vi "VM_ProjetoV5.3.vi"() -> ()   [LabVIEW 2016, in "Projeto_Modbus_Finalizado.lvlib"]
uses:
  Projeto_Modbus_Finalizado.lvlib
  <vilib>/userdefined/High Color/IMAQdx.ctl
  <vilib>/Analysis/baseanly.llb/Mean (DBL).vi
  <vilib>/lvdsc/process/Deploy Library.vi
  <vilib>/Utility/file.llb/Read Delimited Spreadsheet (DBL).vi
  <vilib>/Utility/file.llb/Write Delimited Spreadsheet (DBL).vi
  <vilib>/lvdsc/process/Undeploy Library.vi
  <vilib>/vision/driver/NI_Vision_Acquisition_Software.lvlib
  <resource>/objmgr/imaqdx.rc
  <vilib>/Analysis/NI_AALBase.lvlib
  <vilib>/lvdsc/NI_DSC.lvlib
panel:
  in  "Reset Game":bool
  in  "Reset Count":bool
  out "GameOver":bool
  out "y place":dbl
  out "x place":dbl
  out "pick angle":dbl
  out "place angle":dbl
  out "y pick":dbl
  out "x pick":dbl
  in  "Calibração\nRobô":path=path "C:/Users/rodrigorg1/Desktop/Projeto/calibracaoRobo.csv"
  in  "Calibração\nMesa":path=path "C:/Users/rodrigorg1/Desktop/Projeto/calibracaoMesa.csv"
  out "Error Out":errorcluster
  in  "Cut Limit":dbl=65.0 format="%#_13g"
  in  "Confirma":bool
  out "Status":string
  out "Câmera Robo":T1(plugin-control)
  out "Câmera Mesa":T1(plugin-control)
  in  "Começa jogada":bool
  in  "stop":bool
  in  "Source Câmera Robo":T2="S1156978"
  in  "Source Câmera Mesa":T2="cam0"
  out "Dobrao":bool
  out "Passa Vez":bool
  # "x 91\ny 176"
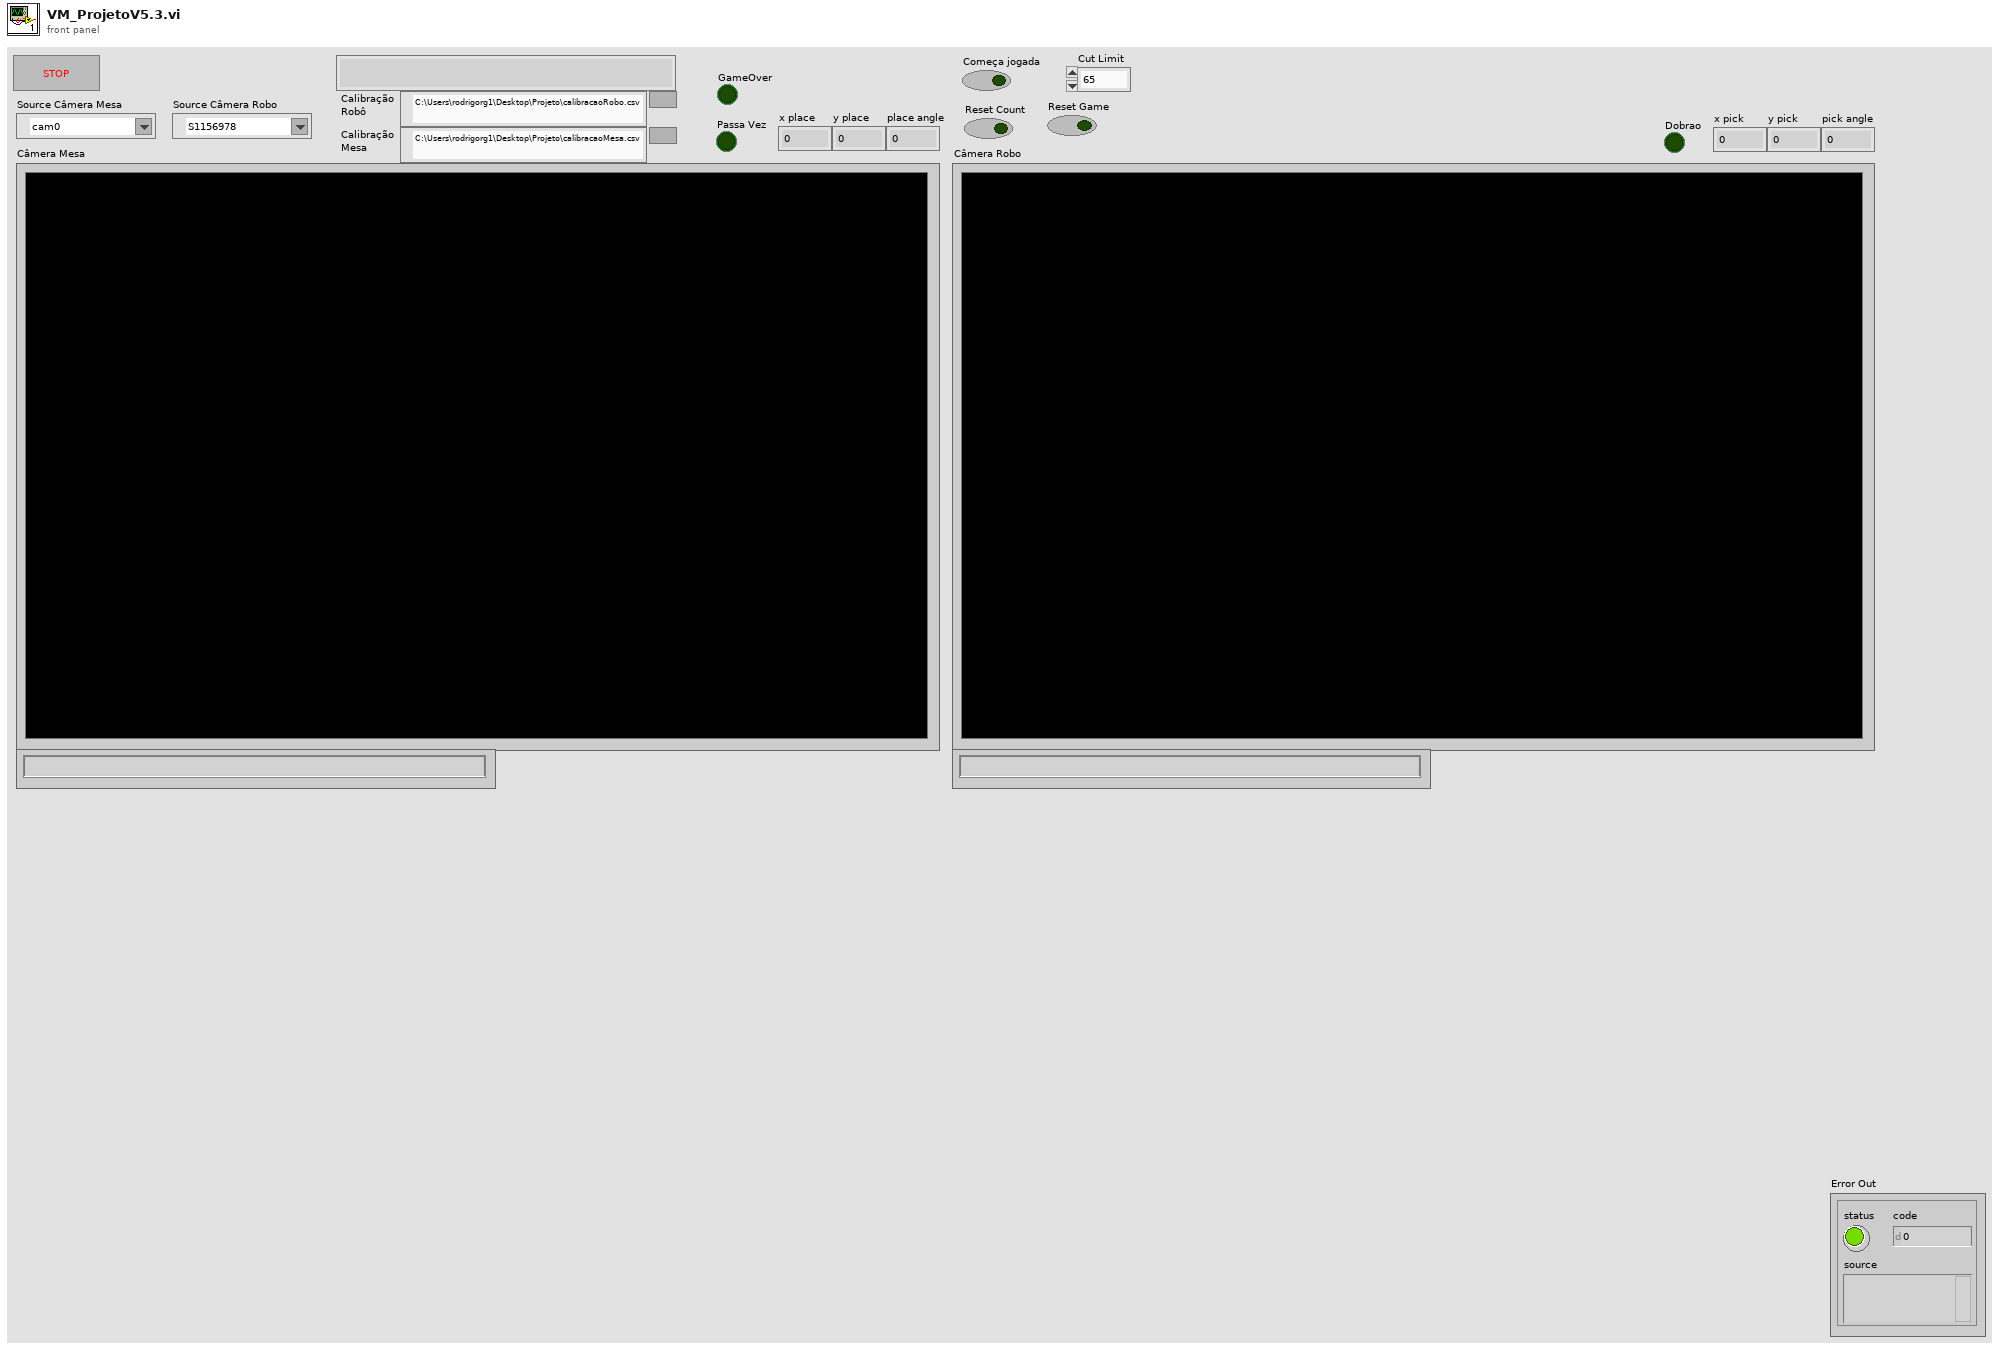
[diagram p1: front panel]
types:
  T1 = typedef "IMAQ Image.ctl" = refnum<image>
  T2 = typedef "IMAQdx.ctl" = refnum<k21>
  T3 = typedef "IMAQ Rectangle" = cluster{"Left":i32, "Top":i32, "Right":i32, "Bottom":i32, "Rotation":dbl}
  T4 = typedef "ROI Descriptor" = cluster{"Global Rectangle":i32[], "Contours":cluster{"ID":enum32{"External", "Internal"}, "Type":u32, "Coordinates":i32[]}[]}
  T5 = cluster{"Position":cluster{"x":sgl, "y":sgl}, "Angle":sgl, "Scale":sgl, "Score":sgl, "Bounding Box":cluster{"x":sgl, "y":sgl}[]}[]
  T6 = cluster{"Centro Peça":dbl[], "Centros Númeors":dbl[][], "Números":u8[], "ROI Números":T4[]}[]
  T7 = cluster{"Centro Peça":dbl[], "Centros Númeors":dbl[][], "Números":u8[], "ROI Números":T4[]}
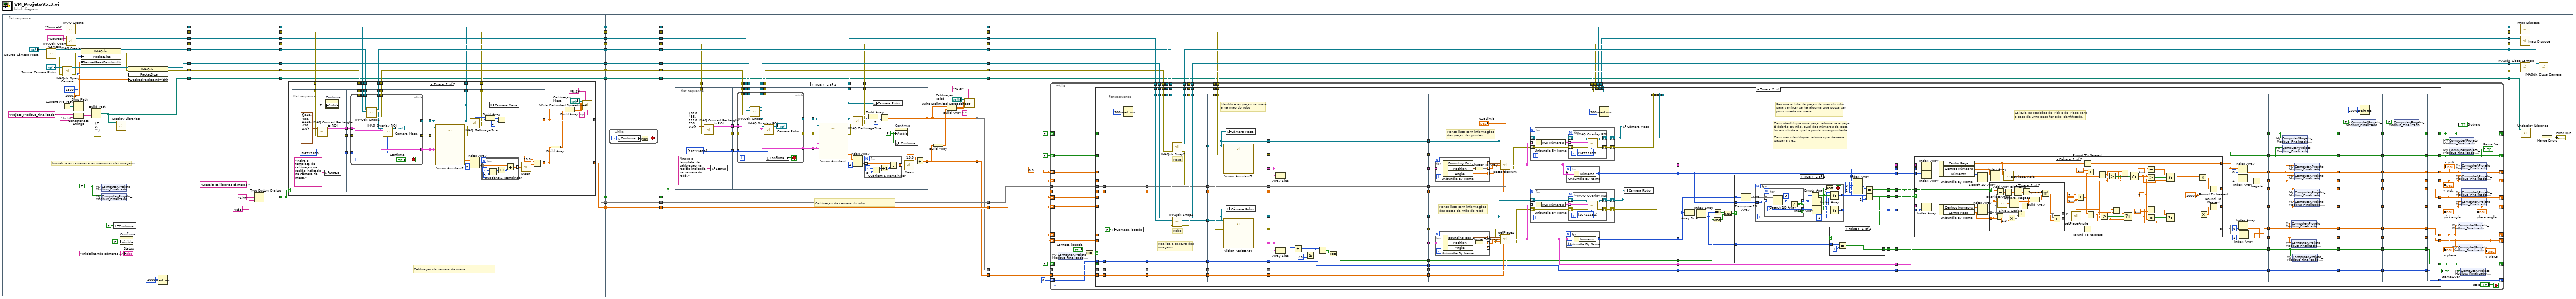
[diagram p0: block diagram]
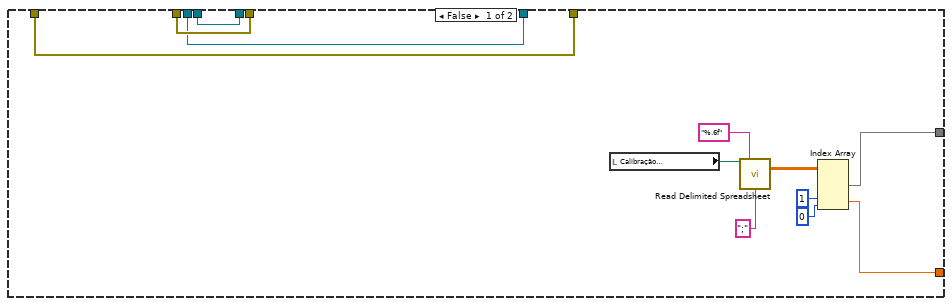
[diagram p2: hidden frame]
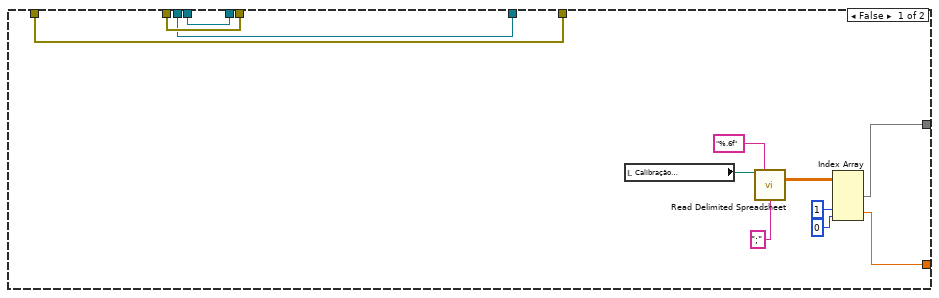
[diagram p3: hidden frame]
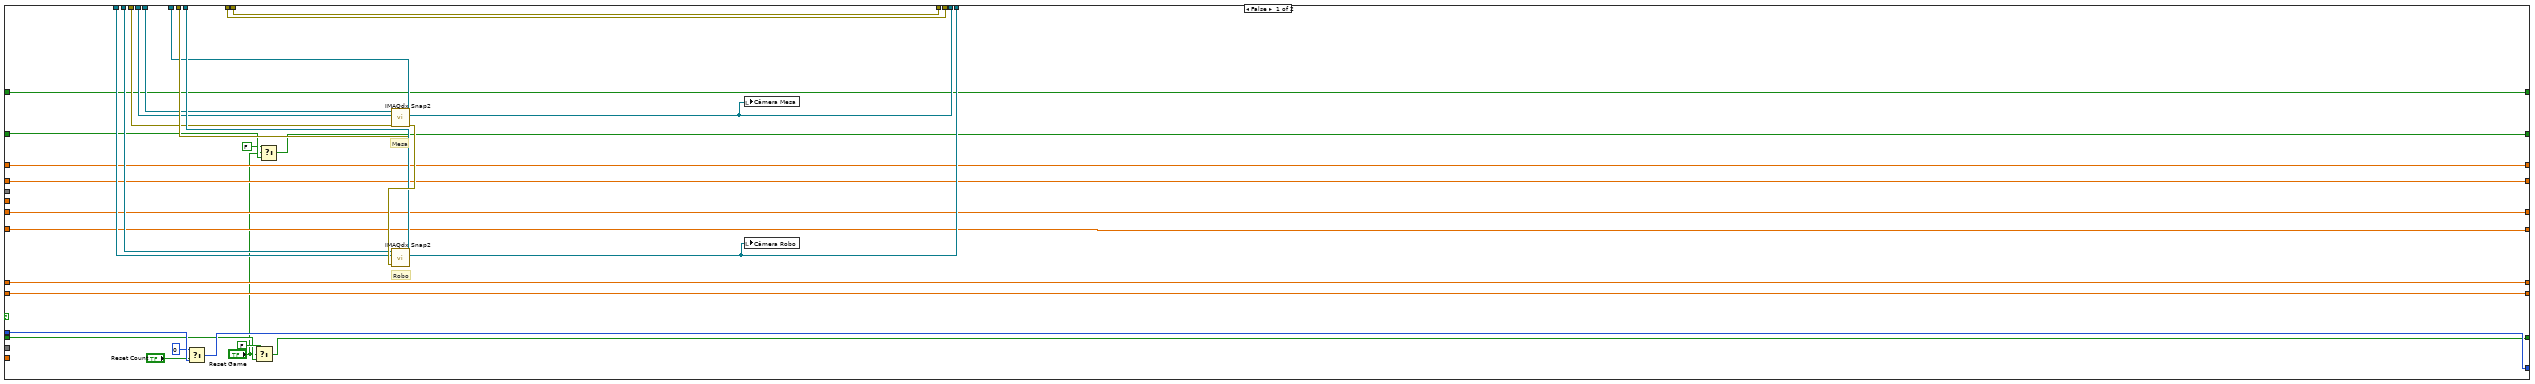
[diagram p4: hidden frame]
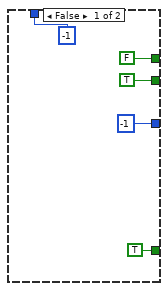
[diagram p5: hidden frame]
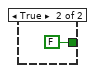
[diagram p6: hidden frame]
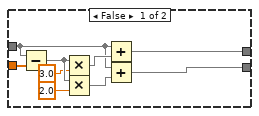
[diagram p7: hidden frame]
diagram:
  n1 = flat-sequence {
    tunnel: [w85] -> w17
    tunnel: [w84] -> w15
    tunnel: [w79] -> w13
    tunnel: [w83] -> w11
    tunnel: [w82] -> w9
    tunnel: [w78] -> w7
    tunnel: [w69] -> w5
    tunnel: [w61] -> w3
    tunnel: w17 -> [w101]
    tunnel: [w101] -> w16
    tunnel: w15 -> [w100]
    tunnel: [w100] -> w14
    tunnel: w13 -> [w99]
    tunnel: [w99] -> w12
    tunnel: w11 -> [w98]
    tunnel: [w98] -> w10
    tunnel: w9 -> [w97]
    tunnel: [w97] -> w8
    tunnel: w7 -> [w96]
    tunnel: [w96] -> w6
    tunnel: w5 -> [w95]
    tunnel: [w95] -> w4
    tunnel: w3 -> [w94]
    tunnel: [w94] -> w2
    tunnel: [w90] -> w1
    tunnel: w16 -> [w115]
    tunnel: w14 -> [w116]
    tunnel: w12 -> [w105]
    tunnel: w10 -> [w114]
    tunnel: w8 -> [w113]
    tunnel: w6 -> [w104]
    tunnel: [w109] -> w41
    tunnel: [w108] -> w39
    tunnel: [w114] -> w37
    tunnel: [w113] -> w35
    tunnel: [w112] -> w33
    tunnel: [w111] -> w31
    tunnel: w4 -> [w111]
    tunnel: [w110] -> w29
    tunnel: [w107] -> w27
    tunnel: [w106] -> w25
    tunnel: [w103] -> w20
    tunnel: w2 -> [w103]
    tunnel: [w102] -> w19
    tunnel: w1 -> [w102]
    tunnel: w41 -> [w213]
    tunnel: [w213] -> w40
    tunnel: w39 -> [w212]
    tunnel: [w212] -> w38
    tunnel: w37 -> [w211]
    tunnel: [w211] -> w36
    tunnel: w35 -> [w210]
    tunnel: [w210] -> w34
    tunnel: w33 -> [w209]
    tunnel: [w209] -> w32
    tunnel: w31 -> [w208]
    tunnel: [w208] -> w30
    tunnel: w29 -> [w207]
    tunnel: [w207] -> w28
    tunnel: w27 -> [w206]
    tunnel: [w206] -> w26
    tunnel: w25 -> [w205]
    tunnel: [w205] -> w24
    tunnel: [w204] -> w21
    tunnel: w20 -> [w204]
    tunnel: w19 -> [w203]
    tunnel: [w203] -> w18
    tunnel: w40 -> [w232]
    tunnel: [w232] -> w52
    tunnel: w38 -> [w231]
    tunnel: [w231] -> w51
    tunnel: w36 -> [w223]
    tunnel: [w222] -> w50
    tunnel: w34 -> [w221]
    tunnel: [w220] -> w49
    tunnel: w32 -> [w230]
    tunnel: [w230] -> w48
    tunnel: w30 -> [w225]
    tunnel: [w224] -> w47
    tunnel: w28 -> [w227]
    tunnel: [w226] -> w46
    tunnel: w26 -> [w229]
    tunnel: [w229] -> w45
    tunnel: w24 -> [w228]
    tunnel: [w228] -> w44
    tunnel: [w219] -> w43
    tunnel: [w218] -> w42
    tunnel: [w217] -> w22
    tunnel: w21 -> [w217]
    tunnel: w18 -> [w216]
    tunnel: [w339] -> w59
    tunnel: [w342] -> w58
    tunnel: [w336] -> w57
    tunnel: [w341] -> w56
    tunnel: [w340] -> w55
    tunnel: [w338] -> w54
    tunnel: [w337] -> w53
    tunnel: w52 -> [w335]
    tunnel: w51 -> [w334]
    tunnel: w50 -> [w333]
    tunnel: w49 -> [w332]
    tunnel: w48 -> [w331]
    tunnel: w47 -> [w330]
    tunnel: w46 -> [w329]
    tunnel: w45 -> [w327]
    tunnel: w44 -> [w328]
    tunnel: w43 -> [w325]
    tunnel: w42 -> [w326]
    tunnel: [w324] -> w23
    tunnel: w22 -> [w324]
    tunnel: w59 -> [w839]
    tunnel: w58 -> [w837]
    tunnel: w57 -> [w841]
    tunnel: w56 -> [w844]
    tunnel: w55 -> [w843]
    tunnel: w54 -> [w840]
    tunnel: w53 -> [w842]
    tunnel: w23 -> [w834]
    frame #0 {
      w60 = FALSE ("000021")
      w73 = 1000.0 ("DesiredPeakBandwidth")
      w74 = u32 1500 ("PacketSize")
      # "Inicializa as câmeras e as memórias das imagens"
      n2 = call <vilib>:"IMAQdx Open Camera.vi"("Session In"="Source Câmera Mesa") -> ("error out"=w77:errorcluster, "Session Out"=w80:T2)  [unwired: 9 in]
      n3 = Current VI's Path() -> (path=w62:path)
      n4 = call <vilib>:"IMAQdx Open Camera.vi"("error in"=w77, "Session In"="Source Câmera Robo") -> ("error out"=w76:errorcluster, "Session Out"=w81:T2)  [unwired: 8 in]
      n5 = call "IMAQ Create"("Image Name"="SourceM") -> ("New Image"=w85:T1, "error out"=w84:errorcluster)  [unwired: 4 in]
      n6 = call "IMAQ Create"("Image Name"="SourceR") -> ("New Image"=w83:T1, "error out"=w82:errorcluster)  [unwired: 4 in]
      n7 = Strip Path(path=w62) -> (stripped path=w63:path)  [unwired: 1 out]
      n8 = Concatenate Strings("Projeto_Modbus_Finalizado" ("library path"), ".lvlib" ("string")) -> (w66:string)
      n9 = property class="IMAQdx"(reference=w80, error in=w76, "PacketSize"=w74, "DesiredPeakBandwidth"=w73) -> (reference out=w79:T2, error out=w75:errorcluster)
      n10 = Build Path(base path=w63, name or relative path=w66) -> (appended path=w61:path)
      n11 = shared-variable "My Computer\\Projeto_Modbus_Finalizado.lvlib\\000021"(w60) -> ()  [unwired: 1 in, 1 out]
      n12 = shared-variable "My Computer\\Projeto_Modbus_Finalizado.lvlib\\000020"(w60) -> ()  [unwired: 1 in, 1 out]
      n13 = local write "Confirma"(FALSE ("Confirma")) -> ()
      n14 = call-poly <vilib>:"Deploy Libraries.vi"("error in (no error)"=errorcluster {"status"=FALSE, "code"=0, "source"=""}, "library path"=w61) -> ()  [unwired: 7 in, 1 out]
      n15 = property on="Confirma" class="Bool (strict)"("Visible"=FALSE) -> ()  [unwired: 2 in, 2 out]
      n16 = property class="IMAQdx"(reference=w81, error in=w75, "PacketSize"=w74, "DesiredPeakBandwidth"=w73) -> (reference out=w69:T2, error out=w78:errorcluster)
      n17 = Wait (ms)(milliseconds to wait=u32 2000) -> ()  [unwired: 1 out]
      "Status" <- "Inicializando câmeras ..." ("Status")
    }
    frame #1 {
      n18 = Two Button Dialog(message="Deseja calibrar as câmeras?", 1:"Não" ("F button name (\"Cancel\")"), 2:"Sim" ("T button name (\"OK\")")) -> (T button?=w90:bool)
    }
    frame #2 {
      # "Calibração da câmera da mesa"
      n19 = case shown="True" w102 {
        tunnel: w116 -> [w125 w143]
        tunnel: w115 -> [w126 w142]
        tunnel: [w127 w141] -> w112
        tunnel: [w128 w140] -> w110
        tunnel: [w126 w139] -> w109
        tunnel: [w125 w138] -> w108
        tunnel: [w118 w133] -> w107
        tunnel: [w117 w134] -> w106
        tunnel: w105 -> [w127 w137]
        tunnel: w104 -> [w128 w136]
        frame False {
          n20 = local read "Calibração\nMesa"() -> (w124:path)
          n21 = call-poly <vilib>:"Read Delimited Spreadsheet.vi"("file path (dialog if empty)"=w124, "format (%.3f)"="%.6f", "delimiter (\\t)"=";" ("delimiter (\\t)")) -> ("all rows"=w121:dbl[][])  [unwired: 7 in, 5 out]
          n22 = Index Array(array=w121, index (row) #2=1, index (col) #2=0) -> (element #1=w117:dbl[], element #2=w118:dbl)  [unwired: 2 in]
        }
        frame True {
          n23 = flat-sequence {
            tunnel: w143 -> [w154]
            tunnel: [w152] -> w149
            tunnel: [w151] -> w148
            tunnel: [u32[] [16711680] ("Colors (Green)")] -> w147
            tunnel: w137 -> [w167]
            tunnel: w136 -> [w166]
            tunnel: w142 -> [w165]
            tunnel: [w164] -> w141
            tunnel: [w163] -> w140
            tunnel: w149 -> [w162]
            tunnel: w148 -> [w161]
            tunnel: [w160] -> w146
            tunnel: [w159] -> w145
            tunnel: [w158] -> w144
            tunnel: w147 -> [w157]
            tunnel: w146 -> [w196]
            tunnel: w145 -> [w195]
            tunnel: [w187] -> w133
            tunnel: w144 -> [w180]
            tunnel: [w180] -> w139
            tunnel: [w182] -> w138
            tunnel: [w181] -> w134
            frame #0 {
              n24 = call "IMAQ Convert Rectangle to ROI"("error in (no error)"=w154, "Rectangle"=T3 {"Left"=818, "Top"=458, "Right"=1118, "Bottom"=758, "Rotation"=0.0}) -> ("error out"=w152:errorcluster, "ROI Descriptor"=w151:T4)  [unwired: 7 in]
              n25 = local write "Status"("Insira o template de calibração na região indicada na câmera da mesa." ("Status")) -> ()
              n26 = property on="Confirma" class="Bool (strict)"("Visible"=TRUE) -> ()  [unwired: 2 in, 2 out]
            }
            frame #1 {
              n27 = while {
                tunnel: w167 -> [w178]
                tunnel: w166 -> [w177]
                tunnel: w165 -> [w176]
                tunnel: [w175] -> w164
                tunnel: [w174] -> w163
                tunnel: w162 -> [w168]
                tunnel: w161 -> [w171]
                tunnel: [w173] -> w160
                tunnel: [w171] -> w159
                tunnel: [w169] -> w158
                tunnel: w157 -> [w170]
                stop <- "Confirma" stop-if-true
                n28 = call <vilib>:"IMAQdx Snap2.vi"("error in"=w177, "Image In"=w176, "Session In"=w178) -> ("error out"=w174:errorcluster, "Image Out"=w169:T1, "Session Out"=w175:T2)  [unwired: 6 in]
                n29 = call "IMAQ Overlay ROI"("Colors (Green)"=w170, "error in (no error)"=w168, "ROI Descriptor"=w171, "Image"=w169) -> ("error out"=w173:errorcluster, "Image Out"=→"Câmera Mesa":T1)  [unwired: 6 in]
              }
            }
            frame #2 {
              n30 = call "Vision Assistant2"("Image In"=w180, "ROI Descriptor (Adv. Straight Edge 1)"=w195, "ROI Descriptor (Copy of Adv. Straight Edge 1)"=w195, "error in"=w196) -> ("Caliper Results (Caliper 2)"=w194:sgl[][], "error out"=w188:errorcluster)  [unwired: 21 in, 1 out]
              n31 = call "IMAQ GetImageSize"("Image"=w180, "error in (no error)"=w188) -> ("Y Resolution"=w186:i32, "X Resolution"=w185:i32, "error out"=w182:errorcluster)  [unwired: 2 in]
              n32 = Index Array(array=w194, index (col)=2 ("disabled index (col)")) -> (element=w192:sgl[])  [unwired: 1 in]
              n33 = for {
                tunnel: w192 -> [w199] mode=indexing
                tunnel: [w197] -> w191 mode=indexing
                i -> [w202]
                n34 = Quotient & Remainder(x=w202, y=5) -> (x-y*floor(x/y)=w200:i32)  [unwired: 1 out]
                n35 = Increment(x=w200) -> (x+1=w198:i32)
                n36 = Divide(x=w199, y=w198) -> (x/y=w197:sgl)
              }
              n37 = Build Array(w185, w186) -> (w184:i32[])
              n38 = local write "Câmera Mesa"(w180) -> ()
              n39 = Divide(x=w184, y=2) -> (x/y=w181:dbl[])
              n40 = call-poly <vilib>:"Mean.vi"("X"=w191) -> ("mean"=w190:dbl)  [unwired: 1 out]
              n41 = Divide(x=10.0, y=w190) -> (x/y=w187:dbl)
            }
          }
          n42 = Build Array(w133) -> (w132:dbl[])
          n43 = Build Array(w134, w132) -> (w131:dbl[][])
          n44 = call-poly <vilib>:"Write Delimited Spreadsheet.vi"("file path (dialog if empty)"="Calibração\nMesa", "format (%.3f)"="%.6f", "2D data"=w131, "delimiter (\\t)"=";" ("delimiter (\\t)")) -> ()  [unwired: 10 in, 2 out]
        }
      }
    }
    frame #3 {
      n45 = while {
        stop <- w215 stop-if-true
        n46 = local read "Confirma"() -> (w214:bool)
        n47 = Not(x=w214) -> (.not. x?=w215:bool)
      }
    }
    frame #4 {
      # "Calibração da câmera do robô"
      n48 = case shown="True" w216 {
        tunnel: w227 -> [w243 w259]
        tunnel: [w243 w258] -> w226
        tunnel: w225 -> [w244 w257]
        tunnel: [w244 w256] -> w224
        tunnel: w223 -> [w242 w255]
        tunnel: [w242 w254] -> w222
        tunnel: w221 -> [w241 w253]
        tunnel: [w241 w252] -> w220
        tunnel: [w233 w246] -> w219
        tunnel: [w234 w245] -> w218
        frame False {
          n49 = local read "Calibração\nRobô"() -> (w235:path)
          n50 = call-poly <vilib>:"Read Delimited Spreadsheet.vi"("file path (dialog if empty)"=w235, "format (%.3f)"="%.6f", "delimiter (\\t)"=";" ("delimiter (\\t)")) -> ("all rows"=w238:dbl[][])  [unwired: 7 in, 5 out]
          n51 = Index Array(array=w238, index (row) #2=1, index (col) #2=0) -> (element #1=w234:dbl[], element #2=w233:dbl)  [unwired: 2 in]
        }
        frame True {
          n52 = flat-sequence {
            tunnel: w253 -> [w270]
            tunnel: [w269] -> w265
            tunnel: [w268] -> w264
            tunnel: [u32[] [16711680] ("Colors (Green)")] -> w263
            tunnel: w257 -> [w282]
            tunnel: w259 -> [w281]
            tunnel: w255 -> [w280]
            tunnel: [w279] -> w256
            tunnel: [w278] -> w258
            tunnel: w265 -> [w277]
            tunnel: w264 -> [w276]
            tunnel: [w275] -> w262
            tunnel: [w274] -> w261
            tunnel: [w273] -> w260
            tunnel: w263 -> [w272]
            tunnel: w262 -> [w312]
            tunnel: w261 -> [w311]
            tunnel: [w303] -> w246
            tunnel: w260 -> [w296]
            tunnel: [w296] -> w254
            tunnel: [w298] -> w252
            tunnel: [w297] -> w245
            frame #0 {
              n53 = call "IMAQ Convert Rectangle to ROI"("error in (no error)"=w270, "Rectangle"=T3 {"Left"=818, "Top"=458, "Right"=1118, "Bottom"=758, "Rotation"=0.0}) -> ("error out"=w269:errorcluster, "ROI Descriptor"=w268:T4)  [unwired: 7 in]
              n54 = local write "Status"("Insira o template de calibração na região indicada na câmera do robô." ("Status")) -> ()
            }
            frame #1 {
              n55 = while {
                tunnel: w282 -> [w294]
                tunnel: w281 -> [w293]
                tunnel: w280 -> [w292]
                tunnel: [w291] -> w279
                tunnel: [w290] -> w278
                tunnel: w277 -> [w289]
                tunnel: w276 -> [w287]
                tunnel: [w288] -> w275
                tunnel: [w287] -> w274
                tunnel: [w286] -> w273
                tunnel: w272 -> [w285]
                stop <- w283 stop-if-true
                n56 = call <vilib>:"IMAQdx Snap2.vi"("error in"=w293, "Image In"=w292, "Session In"=w294) -> ("error out"=w290:errorcluster, "Image Out"=w286:T1, "Session Out"=w291:T2)  [unwired: 6 in]
                n57 = call "IMAQ Overlay ROI"("Colors (Green)"=w285, "error in (no error)"=w289, "ROI Descriptor"=w287, "Image"=w286) -> ("error out"=w288:errorcluster, "Image Out"=→"Câmera Robo":T1)  [unwired: 6 in]
                n58 = local read "Confirma"() -> (w283:bool)
              }
            }
            frame #2 {
              w295 = FALSE ("Visible")
              n59 = call "Vision Assistant"("Image In"=w296, "ROI Descriptor (Adv. Straight Edge 1)"=w311, "ROI Descriptor (Copy of Adv. Straight Edge 1)"=w311, "error in"=w312) -> ("Caliper Results (Caliper 2)"=w310:sgl[][], "error out"=w304:errorcluster)  [unwired: 21 in, 1 out]
              n60 = call "IMAQ GetImageSize"("Image"=w296, "error in (no error)"=w304) -> ("Y Resolution"=w302:i32, "X Resolution"=w301:i32, "error out"=w298:errorcluster)  [unwired: 2 in]
              n61 = Index Array(array=w310, index (col)=2 ("disabled index (col)")) -> (element=w308:sgl[])  [unwired: 1 in]
              n62 = for {
                tunnel: w308 -> [w315] mode=indexing
                tunnel: [w313] -> w307 mode=indexing
                i -> [w318]
                n63 = Quotient & Remainder(x=w318, y=5) -> (x-y*floor(x/y)=w316:i32)  [unwired: 1 out]
                n64 = Increment(x=w316) -> (x+1=w314:i32)
                n65 = Divide(x=w315, y=w314) -> (x/y=w313:sgl)
              }
              n66 = Build Array(w301, w302) -> (w300:i32[])
              n67 = local write "Câmera Robo"(w296) -> ()
              n68 = Divide(x=w300, y=2) -> (x/y=w297:dbl[])
              n69 = property on="Confirma" class="Bool (strict)"("Visible"=w295) -> ()  [unwired: 2 in, 2 out]
              n70 = local write "Confirma"(w295) -> ()
              n71 = call-poly <vilib>:"Mean.vi"("X"=w307) -> ("mean"=w306:dbl)  [unwired: 1 out]
              n72 = Divide(x=10.0, y=w306) -> (x/y=w303:dbl)
            }
          }
          n73 = Build Array(w246) -> (w250:dbl[])
          n74 = Build Array(w245, w250) -> (w249:dbl[][])
          n75 = call-poly <vilib>:"Write Delimited Spreadsheet.vi"("file path (dialog if empty)"="Calibração\nRobô", "format (%.3f)"="%.6f", "2D data"=w249, "delimiter (\\t)"=";" ("delimiter (\\t)")) -> ()  [unwired: 10 in, 2 out]
        }
      }
    }
    frame #5 {
      w321 = 0.0 ("Numeric")
      n76 = while {
        tunnel: w331 -> [w384]
        tunnel: w335 -> [w383]
        tunnel: w333 -> [w382]
        tunnel: w330 -> [w381]
        tunnel: w329 -> [w380]
        tunnel: [w379] -> w342
        tunnel: [w378] -> w341
        tunnel: [w377] -> w340
        tunnel: w334 -> [w376]
        tunnel: w332 -> [w375]
        tunnel: [w374] -> w339
        tunnel: [w373] -> w336
        tunnel: [w371] -> w338
        tunnel: [w370] -> w337
        tunnel: w328 -> [w369]
        tunnel: w327 -> [w368]
        tunnel: w326 -> [w367]
        tunnel: w325 -> [w366]
        shift-right: [w347] -> _
        shift-left: FALSE -> [w355]
        shift-right: [w348] -> _
        shift-left: FALSE -> [w356]
        shift-right: [w362] -> _
        shift-left: w321 -> [w354]
        shift-right: [w361] -> _
        shift-left: w321 -> [w353]
        shift-right: [w360] -> _
        shift-left: w321 -> [w352]
        shift-right: [w359] -> _
        shift-left: w321 -> [w351]
        shift-right: [w358] -> _
        shift-left: w321 -> [w350]
        shift-right: [w357] -> _
        shift-left: w321 -> [w349]
        shift-right: [w343] -> _
        shift-left: FALSE -> [w346]
        shift-right: [w344] -> _
        shift-left: 0 ("y") -> [w345]
        stop <- "stop" stop-if-true
        n77 = shared-variable "My Computer\\Projeto_Modbus_Finalizado.lvlib\\000022"() -> (w363:bool)  [unwired: 1 in, 1 out]
        n78 = Or(x="Começa jogada", y=w363) -> (x .or. y?=w365:bool)
        n79 = case shown="True" w365 {
          tunnel: w384 -> [w406 w524]
          tunnel: w383 -> [w405 w523]
          tunnel: w382 -> [w412 w522]
          tunnel: w381 -> [w411 w521]
          tunnel: w380 -> [w408 w520]
          tunnel: [w407 w519] -> w379
          tunnel: [w410 w518] -> w378
          tunnel: [w409 w517] -> w377
          tunnel: w376 -> [w415 w515]
          tunnel: w375 -> [w414 w513]
          tunnel: [w404 w493] -> w374
          tunnel: [w403 w494] -> w373
          tunnel: [w415 w491] -> w371
          tunnel: [w414 w492] -> w370
          tunnel: w369 -> [_ w484]
          tunnel: w368 -> [_ w501]
          tunnel: w367 -> [_ w475]
          tunnel: w366 -> [_ w473]
          tunnel: [w401 w490] -> w362
          tunnel: [w399 w489] -> w361
          tunnel: [w400 w488] -> w360
          tunnel: [w398 w487] -> w359
          tunnel: [w397 w486] -> w358
          tunnel: [w396 w485] -> w357
          tunnel: [w387 w439] -> w347
          tunnel: [w402 w438] -> w348
          tunnel: w356 -> [w402 _]
          tunnel: w355 -> [w388 _]
          tunnel: w354 -> [w401 _]
          tunnel: w353 -> [w399 _]
          tunnel: w352 -> [w400 _]
          tunnel: w351 -> [w398 _]
          tunnel: w350 -> [w397 _]
          tunnel: w349 -> [w396 _]
          tunnel: [w389 w417] -> w343
          tunnel: w346 -> [w390 _]
          tunnel: w345 -> [w395 w447]
          tunnel: [w394 w416] -> w344
          frame False {
            # "Robo"
            # "Mesa"
            n80 = Select(t=0, s="Reset Count", f=w395) -> (s? t:f=w394:i32)
            n81 = Select(t=FALSE, s="Reset Game", f=w390) -> (s? t:f=w389:bool)
            n82 = Select(t=FALSE, s="Reset Game", f=w388) -> (s? t:f=w387:bool)
            n83 = call <vilib>:"IMAQdx Snap2.vi"("error in"=w408, "Image In"=w405, "Session In"=w406) -> ("error out"=w413:errorcluster, "Image Out"=w404:T1, "Session Out"=w407:T2)  [unwired: 6 in]
            n84 = call <vilib>:"IMAQdx Snap2.vi"("error in"=w413, "Image In"=w412, "Session In"=w411) -> ("error out"=w409:errorcluster, "Image Out"=w403:T1, "Session Out"=w410:T2)  [unwired: 6 in]
            n85 = local write "Câmera Mesa"(w404) -> ()
            n86 = local write "Câmera Robo"(w403) -> ()
          }
          frame True {
            n87 = flat-sequence {
              tunnel: w501 -> [w530]
              tunnel: w484 -> [w531]
              tunnel: [w531] -> w496
              tunnel: [w530] -> w495
              tunnel: w475 -> [w528]
              tunnel: [w528] -> w474
              tunnel: w473 -> [w527]
              tunnel: [w527] -> w472
              tunnel: w447 -> [w526]
              tunnel: [w526] -> w444
              tunnel: w524 -> [w547]
              tunnel: w523 -> [w546]
              tunnel: w522 -> [w545]
              tunnel: w521 -> [w544]
              tunnel: w520 -> [w538]
              tunnel: [w543] -> w519
              tunnel: [w542] -> w518
              tunnel: [w541] -> w517
              tunnel: [w540] -> w516
              tunnel: [w539] -> w514
              tunnel: [w536] -> w500
              tunnel: [w535] -> w499
              tunnel: [w534] -> w498
              tunnel: [w533] -> w497
              tunnel: w496 -> [w536]
              tunnel: w495 -> [w535]
              tunnel: w474 -> [w534]
              tunnel: w472 -> [w533]
              tunnel: [w532] -> w445
              tunnel: w444 -> [w532]
              tunnel: w516 -> [w550]
              tunnel: w515 -> [w560]
              tunnel: w514 -> [w549]
              tunnel: w513 -> [w559]
              tunnel: [w558] -> w471
              tunnel: [w557] -> w469
              tunnel: [w549] -> w467
              tunnel: [w550] -> w465
              tunnel: [w556] -> w463
              tunnel: [w555] -> w461
              tunnel: [w554] -> w459
              tunnel: w500 -> [w554]
              tunnel: [w553] -> w457
              tunnel: w499 -> [w553]
              tunnel: [w552] -> w455
              tunnel: w498 -> [w552]
              tunnel: w497 -> [w551]
              tunnel: [w551] -> w453
              tunnel: [w548] -> w446
              tunnel: w445 -> [w548]
              tunnel: w471 -> [w569]
              tunnel: [w569] -> w470
              tunnel: w469 -> [w570]
              tunnel: [w570] -> w468
              tunnel: w467 -> [w578]
              tunnel: [w578] -> w466
              tunnel: w465 -> [w577]
              tunnel: [w577] -> w464
              tunnel: w463 -> [w576]
              tunnel: [w576] -> w462
              tunnel: w461 -> [w575]
              tunnel: [w575] -> w460
              tunnel: w459 -> [w574]
              tunnel: [w574] -> w458
              tunnel: w457 -> [w573]
              tunnel: [w573] -> w456
              tunnel: w455 -> [w572]
              tunnel: [w572] -> w454
              tunnel: w453 -> [w571]
              tunnel: [w571] -> w452
              tunnel: [w563] -> w451
              tunnel: w446 -> [w562]
              tunnel: [w561] -> w440
              tunnel: w470 -> [w608]
              tunnel: w468 -> [w607]
              tunnel: w466 -> [w582]
              tunnel: w464 -> [w583]
              tunnel: w462 -> [w603]
              tunnel: w460 -> [w599]
              tunnel: [w598] -> w512
              tunnel: [w597] -> w511
              tunnel: [w591] -> w510
              tunnel: [w589] -> w509
              tunnel: w458 -> [w596]
              tunnel: w456 -> [w595]
              tunnel: w454 -> [w594]
              tunnel: w452 -> [w593]
              tunnel: [w584] -> w494
              tunnel: [w587] -> w492
              tunnel: [w585] -> w493
              tunnel: [w586] -> w491
              tunnel: w451 -> [w580]
              tunnel: [w580] -> w450
              tunnel: [w579] -> w443
              tunnel: w440 -> [w579]
              tunnel: w512 -> [w656]
              tunnel: w511 -> [w655]
              tunnel: w510 -> [w662]
              tunnel: w509 -> [w658]
              tunnel: [w662] -> w508
              tunnel: [w661] -> w507
              tunnel: [w660] -> w506
              tunnel: [w659] -> w505
              tunnel: [w658] -> w504
              tunnel: [w657] -> w503
              tunnel: [w656] -> w502
              tunnel: w450 -> [w651]
              tunnel: [w650] -> w448
              tunnel: w443 -> [w649]
              tunnel: [w649] -> w442
              tunnel: w508 -> [w721]
              tunnel: w507 -> [w711]
              tunnel: w506 -> [w712]
              tunnel: w505 -> [w724]
              tunnel: w504 -> [w720]
              tunnel: w503 -> [w723]
              tunnel: w502 -> [w722]
              tunnel: [w713] -> w437
              tunnel: [w705] -> w435
              tunnel: [w710] -> w433
              tunnel: [w709] -> w431
              tunnel: [w707] -> w429
              tunnel: [w708] -> w427
              tunnel: [w712] -> w425
              tunnel: [w711] -> w423
              tunnel: [w704] -> w421
              tunnel: w448 -> [w704]
              tunnel: w442 -> [w703]
              tunnel: [w703] -> w419
              tunnel: w437 -> [w807]
              tunnel: [w807] -> w436
              tunnel: w435 -> [w806]
              tunnel: [w806] -> w434
              tunnel: w433 -> [w805]
              tunnel: [w805] -> w432
              tunnel: w431 -> [w804]
              tunnel: [w804] -> w430
              tunnel: w429 -> [w803]
              tunnel: [w803] -> w428
              tunnel: w427 -> [w802]
              tunnel: [w802] -> w426
              tunnel: w425 -> [w808]
              tunnel: [w808] -> w424
              tunnel: w423 -> [w809]
              tunnel: [w809] -> w422
              tunnel: w421 -> [w801]
              tunnel: [w801] -> w420
              tunnel: w419 -> [w810]
              tunnel: [w810] -> w418
              tunnel: w436 -> [w822]
              tunnel: w434 -> [w821]
              tunnel: w432 -> [w820]
              tunnel: w430 -> [w819]
              tunnel: w428 -> [w818]
              tunnel: w426 -> [w817]
              tunnel: w424 -> [w816]
              tunnel: w422 -> [w815]
              tunnel: [w822] -> w483
              tunnel: [w821] -> w482
              tunnel: [w820] -> w481
              tunnel: [w819] -> w480
              tunnel: [w818] -> w479
              tunnel: [w817] -> w478
              tunnel: [w816] -> w477
              tunnel: [w815] -> w476
              tunnel: [w812] -> w449
              tunnel: w420 -> [w812]
              tunnel: [w811] -> w441
              tunnel: w418 -> [w811]
              tunnel: [w826] -> w438
              tunnel: [w827] -> w439
              tunnel: [w828] -> w485
              tunnel: [w829] -> w486
              tunnel: [w830] -> w487
              tunnel: [w831] -> w488
              tunnel: [w832] -> w489
              tunnel: [w833] -> w490
              tunnel: w483 -> [w833]
              tunnel: w482 -> [w832]
              tunnel: w481 -> [w831]
              tunnel: w480 -> [w830]
              tunnel: w479 -> [w829]
              tunnel: w478 -> [w828]
              tunnel: w477 -> [w827]
              tunnel: w476 -> [w826]
              tunnel: [w824] -> w417
              tunnel: w449 -> [w824]
              tunnel: [w823] -> w416
              tunnel: w441 -> [w823]
              frame #0 {
                n88 = local write "Começa jogada"(FALSE ("Começa jogada")) -> ()
                n89 = Wait (ms)(milliseconds to wait=u32 500) -> ()  [unwired: 1 out]
              }
              frame #1 {
                # "Realiza a captura das\nimagens"
                # "Robo"
                # "Mesa"
                n90 = call <vilib>:"IMAQdx Snap2.vi"("error in"=w538, "Image In"=w546, "Session In"=w547) -> ("error out"=w537:errorcluster, "Image Out"=w540:T1, "Session Out"=w543:T2)  [unwired: 6 in]
                n91 = call <vilib>:"IMAQdx Snap2.vi"("error in"=w537, "Image In"=w545, "Session In"=w544) -> ("error out"=w541:errorcluster, "Image Out"=w539:T1, "Session Out"=w542:T2)  [unwired: 6 in]
              }
              frame #2 {
                # "Identifica as peças na mesa\ne na mão do robô"
                n92 = call "Vision Assistant3"("Image In"=w550, "error in"=w560) -> ("Matches (Pattern Matching 1)"=w557:T5, "error out"=w556:errorcluster)  [unwired: 23 in, 1 out]
                n93 = call "Vision Assistant4"("Image In"=w549, "error in"=w559) -> ("Matches (Pattern Matching 1)"=w558:T5, "error out"=w555:errorcluster)  [unwired: 23 in, 1 out]
                n94 = local write "Câmera Mesa"(w550) -> ()
                n95 = local write "Câmera Robo"(w549) -> ()
              }
              frame #3 {
                n96 = Array Size(array=w570) -> (size(s)=w568:i32)
                n97 = Array Size(array=w569) -> (size(s)=w567:i32)
                n98 = Add(x=w568, y=w567) -> (x+y=w561:i32)
                n99 = Greater Or Equal?(x=w561, y=28) -> (x >= y?=w564:bool)
                n100 = Equal?(x=w561, y=w562) -> (x = y?=w565:bool)
                n101 = Or(x=w565, y=w564) -> (x .or. y?=w563:bool)
              }
              frame #4 {
                # "Monta lista com informações\ndas peças das pontas"
                # "Monta lista com informações\ndas peças da mão do robô"
                n102 = for {
                  tunnel: w607 -> [w641] mode=indexing
                  tunnel: [w639] -> w605 mode=indexing
                  tunnel: [w638] -> w606 mode=indexing
                  tunnel: [w637] -> w604 mode=indexing
                  n103 = Unbundle By Name(w641) -> ("Bounding Box"=w638:cluster{"x":sgl, "y":sgl}[], "Position"=w640:cluster{"x":sgl, "y":sgl}, "Angle"=w637:sgl)
                  n104 = Cluster To Array(cluster=w640) -> (array=w639:sgl[])
                }
                n105 = for {
                  tunnel: w608 -> [w646] mode=indexing
                  tunnel: [w644] -> w601 mode=indexing
                  tunnel: [w643] -> w602 mode=indexing
                  tunnel: [w642] -> w600 mode=indexing
                  n106 = Unbundle By Name(w646) -> ("Bounding Box"=w643:cluster{"x":sgl, "y":sgl}[], "Position"=w645:cluster{"x":sgl, "y":sgl}, "Angle"=w642:sgl)
                  n107 = Cluster To Array(cluster=w645) -> (array=w644:sgl[])
                }
                n108 = call "getBorderNum.vi"("Refnum in"=w583, "Cut Limit"="Cut Limit", "Bounding Box"=w606, "Position"=w605, "Angle"=w604, "error in (no error)"=w603, "Step"=w595, "Origin Pixel"=w596) -> ("Data Pieces"=w591:T6, "error out"=w590:errorcluster)  [unwired: 5 in, 1 out]
                n109 = call "getPieces.vi"("Refnum in"=w582, "Bounding Box"=w602, "Position"=w601, "Angle"=w600, "error in (no error)"=w599, "Step"=w593, "Origin Pixel"=w594) -> ("Data Pieces"=w589:T6, "error out"=w588:errorcluster)  [unwired: 6 in, 1 out]
                n110 = for {
                  tunnel: w591 -> [w626] mode=indexing
                  shift-right: [w623] -> w585
                  shift-left: w583 -> [w624]
                  shift-right: [w621] -> w586
                  shift-left: w590 -> [w622]
                  n111 = Unbundle By Name(w626) -> ("ROI Números"=w625:T4[])
                  n112 = for {
                    tunnel: w625 -> [w632] mode=indexing
                    shift-right: [w630] -> w623
                    shift-left: w624 -> [w631]
                    shift-right: [w628] -> w621
                    shift-left: w622 -> [w629]
                    n113 = call "IMAQ Overlay ROI"("Colors (Green)"=u32[] [16711680], "error in (no error)"=w629, "ROI Descriptor"=w632, "Image"=w631) -> ("error out"=w628:errorcluster, "Image Out"=w630:T1)  [unwired: 6 in]
                  }
                }
                n114 = for {
                  tunnel: w589 -> [w614] mode=indexing
                  shift-right: [w611] -> w584
                  shift-left: w582 -> [w612]
                  shift-right: [w609] -> w587
                  shift-left: w588 -> [w610]
                  n115 = Unbundle By Name(w614) -> ("ROI Números"=w613:T4[])
                  n116 = for {
                    tunnel: w613 -> [w620] mode=indexing
                    shift-right: [w618] -> w611
                    shift-left: w612 -> [w619]
                    shift-right: [w616] -> w609
                    shift-left: w610 -> [w617]
                    n117 = call "IMAQ Overlay ROI"("Colors (Green)"=u32[] [16711680], "error in (no error)"=w617, "ROI Descriptor"=w620, "Image"=w619) -> ("error out"=w616:errorcluster, "Image Out"=w618:T1)  [unwired: 6 in]
                  }
                }
                n118 = for {
                  tunnel: w591 -> [w636] mode=indexing
                  tunnel: [w635] -> w598 mode=concatenating
                  n119 = Unbundle By Name(w636) -> ("Números"=w635:u8[])
                }
                n120 = for {
                  tunnel: w589 -> [w634] mode=indexing
                  tunnel: [w633] -> w597 mode=indexing
                  n121 = Unbundle By Name(w634) -> ("Números"=w633:u8[])
                }
                n122 = Wait (ms)(milliseconds to wait=u32 500) -> ()  [unwired: 1 out]
                n123 = local write "Câmera Mesa"(w585) -> ()
                n124 = local write "Câmera Robo"(w584) -> ()
              }
              frame #5 {
                # "Caso identifique uma peça, retorna se a peça\né dobrão ou não, qual dos números da peça\nfoi escolhida e qual a ponta correspondente.\n\nCaso não identifique, retorna que deve-se\npassar a vez."
                # "Percorre a lista de peças da mão do robô\npara verificar se há alguma que possa ser\nposicionada na mesa"
                n125 = Array Size(array=w655) -> (size(s)=w648:i32[])
                n126 = Index Array(array=w648) -> (element=w647:i32)  [unwired: 1 in]
                n127 = Not(x=w651) -> (.not. x?=w652:bool)
                n128 = Not Equal To 0?(x=w647) -> (x != 0?=w653:bool)
                n129 = And(x=w653, y=w652) -> (x .and. y?=w654:bool)
                n130 = case shown="True" w654 {
                  tunnel: w655 -> [_ w675]
                  tunnel: [FALSE w674] -> w661
                  tunnel: [TRUE w670] -> w660
                  tunnel: [-1 ("t") w673] -> w659
                  tunnel: [-1 ("index of element") w672] -> w657
                  tunnel: w656 -> [_ w671]
                  tunnel: w647 -> [_ w669]
                  tunnel: [TRUE w668] -> w650
                  frame False {
                  }
                  frame True {
                    n131 = Transpose 2D Array(2D array=w675) -> (transposed array=w677:u8[][])
                    n132 = for {
                      tunnel: w677 -> [w696] mode=indexing
                      tunnel: w671 -> [w695]
                      tunnel: [w687] -> w673
                      tunnel: [w686] -> w672
                      stop <- w691 stop-if-true
                      w688 = -1 ("t")
                      n133 = for {
                        tunnel: w696 -> [w702]
                        tunnel: w695 -> [w701] mode=indexing
                        tunnel: [w699] -> w693 mode=indexing if=w697
                        tunnel: [w698] -> w692 mode=indexing if=w697
                        i -> [w698]
                        n134 = Search 1D Array(1D array=w702, element=w701) -> (index of element=w699:i32)  [unwired: 1 in]
                        n135 = Not Equal?(x=w699, y=-1) -> (x != y?=w697:bool)
                      }
                      n136 = Empty Array?(array=w693) -> (empty?=w689:bool)
                      n137 = Index Array(array=w693) -> (element=w694:i32)  [unwired: 1 in]
                      n138 = Index Array(array=w692) -> (element=w690:i32)  [unwired: 1 in]
                      n139 = Not(x=w689) -> (.not. x?=w691:bool)
                      n140 = Select(t=w688, s=w689, f=w694) -> (s? t:f=w686:i32)
                      n141 = Select(t=w688, s=w689, f=w690) -> (s? t:f=w687:i32)
                    }
                    n142 = Index Array(array=w677, index (row) #1=0 ("disabled index (row)"), index (col) #1=w672, index (row) #2=1 ("disabled index (row)"), index (col) #2=w672) -> (element #1=w681:u8, element #2=w680:u8)
                    n143 = Equal?(x=w681, y=w680) -> (x = y?=w674:bool)
                    n144 = Equal?(x=w672, y=-1) -> (x = y?=w670:bool)
                    n145 = case shown="False" w670 {
                      tunnel: w669 -> [w684 _]
                      tunnel: [w682 FALSE] -> w668
                      frame False {
                        n146 = Equal?(x=w684, y=1) -> (x = y?=w682:bool)
                      }
                      frame True {
                      }
                    }
                  }
                }
              }
              frame #6 {
                # "Calcula as posições de Pick e de Place para\no caso de uma peça ter sido identificada."
                n147 = case shown="False" w712 {
                  tunnel: w720 -> [w770 _]
                  tunnel: w723 -> [w769 _]
                  tunnel: w724 -> [w766 _]
                  tunnel: w721 -> [w768 _]
                  tunnel: w722 -> [w758 _]
                  tunnel: w711 -> [w763 _]
                  tunnel: [w756 _] -> w718
                  tunnel: [w755 _] -> w714
                  tunnel: [w751 _] -> w709
                  tunnel: [w752 _] -> w710
                  frame False {
                    w735 = 3.141592653589793
                    w739 = 6.283185307179586
                    w757 = 1000.0
                    n148 = Index Array(array=w770, index=w769) -> (element=w771:T7)
                    n149 = Index Array(array=w758, index=w766) -> (element=w765:u8)
                    n150 = Index Array(array=w768, index=w766) -> (element=w767:T7)
                    n151 = Unbundle By Name(w771) -> ("Centro Peça"=w753:dbl[], "Centros Númeors"=w773:dbl[][], "Números"=w772:u8[])
                    n152 = Unbundle By Name(w767) -> ("Centros Númeors"=w760:dbl[][], "Centro Peça"=w759:dbl[])
                    n153 = Search 1D Array(1D array=w772, element=w765) -> (index of element=w774:i32)  [unwired: 1 in]
                    n154 = Index Array(array=w760) -> (element=w762:dbl[])  [unwired: 2 in]
                    n155 = case shown="True" w763 {
                      tunnel: w762 -> [w778 w793]
                      tunnel: w759 -> [w782 w794]
                      tunnel: [w776 w786] -> w761
                      tunnel: [w775 w785] -> w754
                      frame False {
                        n156 = Subtract(x=w778, y=w782) -> (x-y=w781:dbl[])
                        n157 = Multiply(x=w781, y=3.0) -> (x*y=w783:dbl[])
                        n158 = Multiply(x=w781, y=2.0) -> (x*y=w777:dbl[])
                        n159 = Add(x=w778, y=w783) -> (x+y=w775:dbl[])
                        n160 = Add(x=w778, y=w777) -> (x+y=w776:dbl[])
                      }
                      frame True {
                        n161 = Subtract(x=w793, y=w794) -> (x-y=w800:dbl[])
                        n162 = Subtract(x=w794, y=w793) -> (x-y=w797:dbl[])
                        n163 = call "getPieceAngle.vi"("Center Num"=w793, "Center Piece"=w794) -> ("Angle"=w792:dbl)
                        n164 = Square(x=w797) -> (x^2=w796:dbl[])
                        n165 = Multiply(x=w800, y=2.0) -> (x*y=w798:dbl[])
                        n166 = Sine & Cosine(0:w792) -> (1:w790:dbl, 2:w791:dbl)
                        n167 = Add Array Elements(numeric array=w796) -> (sum=w795:dbl)
                        n168 = Add(x=w793, y=w798) -> (x+y=w785:dbl[])
                        n169 = Negate(x=w791) -> (-x=w789:dbl)
                        n170 = Square Root(x=w795) -> (sqrt(x)=w787:dbl)
                        n171 = Build Array(w789, w790) -> (w788:dbl[])
                        n172 = Multiply(x=w787, y=w788) -> (x*y=w784:dbl[])
                        n173 = Add(x=w785, y=w784) -> (x+y=w786:dbl[])
                      }
                    }
                    n174 = Index Array(array=w773, index (row)=w774) -> (element=w764:dbl[])  [unwired: 1 in]
                    n175 = call "getPieceAngle.vi"("Center Num"=w764, "Center Piece"=w753) -> ("Angle"=w747:dbl)
                    n176 = call "getPieceAngle.vi"("Center Num"=w761, "Center Piece"=w754) -> ("Angle"=w748:dbl)
                    n177 = Add(x=1.5707963267948966, y=w739) -> (x+y=w738:dbl)
                    n178 = Round To Nearest(number=w753) -> (nearest integer value=w756:dbl[])
                    n179 = Round To Nearest(number=w754) -> (nearest integer value=w755:dbl[])
                    n180 = Add(x=1.5707963267948966, y=w738) -> (x+y=w737:dbl)
                    n181 = Subtract(x=w738, y=w748) -> (x-y=w740:dbl)
                    n182 = Subtract(x=w737, y=w747) -> (x-y=w743:dbl)
                    n183 = Greater?(x=w740, y=w739) -> (0:w745:bool)
                    n184 = Greater?(x=w743, y=w739) -> (0:w744:bool)
                    n185 = Subtract(x=w740, y=w739) -> (x-y=w741:dbl)
                    n186 = Subtract(x=w743, y=w739) -> (x-y=w742:dbl)
                    n187 = Select(t=w741, s=w745, f=w740) -> (s? t:f=w729:dbl)
                    n188 = Select(t=w742, s=w744, f=w743) -> (s? t:f=w732:dbl)
                    n189 = Subtract(x=w732, y=6.283185307179586) -> (x-y=w725:dbl)
                    n190 = Greater?(x=w732, y=w735) -> (0:w734:bool)
                    n191 = Subtract(x=w729, y=6.283185307179586) -> (x-y=w728:dbl)
                    n192 = Greater?(x=w729, y=w735) -> (0:w733:bool)
                    n193 = Select(t=w725, s=w734, f=w732) -> (s? t:f=w726:dbl)
                    n194 = Select(t=w728, s=w733, f=w729) -> (s? t:f=w727:dbl)
                    n195 = Multiply(x=w726, y=w757) -> (x*y=w750:dbl)
                    n196 = Multiply(x=w757, y=w727) -> (x*y=w749:dbl)
                    n197 = Round To Nearest(number=w750) -> (nearest integer value=w752:dbl)
                    n198 = Round To Nearest(number=w749) -> (nearest integer value=w751:dbl)
                  }
                  frame True {
                  }
                }
                n199 = Index Array(array=w718, index=0) -> (element=w713:dbl)
                n200 = Index Array(array=w718, index=1) -> (element=w706:dbl)
                n201 = Index Array(array=w714, index=0) -> (element=w708:dbl)
                n202 = Index Array(array=w714, index=1) -> (element=w707:dbl)
                n203 = Negate(x=w706) -> (-x=w705:dbl)
              }
              frame #7 {
                n204 = shared-variable "My Computer\\Projeto_Modbus_Finalizado.lvlib\\000018"(w809) -> ()  [unwired: 1 in, 1 out]
                n205 = shared-variable "My Computer\\Projeto_Modbus_Finalizado.lvlib\\000019"(w808) -> ()  [unwired: 1 in, 1 out]
                n206 = shared-variable "My Computer\\Projeto_Modbus_Finalizado.lvlib\\400131"(w803) -> ()  [unwired: 1 in, 1 out]
                n207 = shared-variable "My Computer\\Projeto_Modbus_Finalizado.lvlib\\400132"(w802) -> ()  [unwired: 1 in, 1 out]
                n208 = shared-variable "My Computer\\Projeto_Modbus_Finalizado.lvlib\\000020"(w801) -> ()  [unwired: 1 in, 1 out]
                n209 = shared-variable "My Computer\\Projeto_Modbus_Finalizado.lvlib\\400130"(w806) -> ()  [unwired: 1 in, 1 out]
                n210 = shared-variable "My Computer\\Projeto_Modbus_Finalizado.lvlib\\400129"(w807) -> ()  [unwired: 1 in, 1 out]
                n211 = shared-variable "My Computer\\Projeto_Modbus_Finalizado.lvlib\\400133"(w805) -> ()  [unwired: 1 in, 1 out]
                n212 = shared-variable "My Computer\\Projeto_Modbus_Finalizado.lvlib\\400134"(w804) -> ()  [unwired: 1 in, 1 out]
              }
              frame #8 {
                n213 = shared-variable "My Computer\\Projeto_Modbus_Finalizado.lvlib\\000021"(TRUE ("000021")) -> ()  [unwired: 1 in, 1 out]
                n214 = Wait (ms)(milliseconds to wait=u32 2000) -> ()  [unwired: 1 out]
              }
              frame #9 {
                n215 = shared-variable "My Computer\\Projeto_Modbus_Finalizado.lvlib\\000021"(FALSE ("000021")) -> ()  [unwired: 1 in, 1 out]
              }
            }
          }
        }
        "Dobrao" <- w348
        "Passa Vez" <- w347
        "x pick" <- w362
        "y pick" <- w361
        "place angle" <- w359
        "pick angle" <- w360
        "x place" <- w358
        "y place" <- w357
        "GameOver" <- w343
        n216 = shared-variable "My Computer\\Projeto_Modbus_Finalizado.lvlib\\000018"(w348) -> ()  [unwired: 1 in, 1 out]
        n217 = shared-variable "My Computer\\Projeto_Modbus_Finalizado.lvlib\\000019"(w347) -> ()  [unwired: 1 in, 1 out]
        n218 = shared-variable "My Computer\\Projeto_Modbus_Finalizado.lvlib\\400131"(w358) -> ()  [unwired: 1 in, 1 out]
        n219 = shared-variable "My Computer\\Projeto_Modbus_Finalizado.lvlib\\400132"(w357) -> ()  [unwired: 1 in, 1 out]
        n220 = shared-variable "My Computer\\Projeto_Modbus_Finalizado.lvlib\\000020"(w343) -> ()  [unwired: 1 in, 1 out]
        n221 = shared-variable "My Computer\\Projeto_Modbus_Finalizado.lvlib\\400130"(w361) -> ()  [unwired: 1 in, 1 out]
        n222 = shared-variable "My Computer\\Projeto_Modbus_Finalizado.lvlib\\400129"(w362) -> ()  [unwired: 1 in, 1 out]
        n223 = shared-variable "My Computer\\Projeto_Modbus_Finalizado.lvlib\\400133"(w360) -> ()  [unwired: 1 in, 1 out]
        n224 = shared-variable "My Computer\\Projeto_Modbus_Finalizado.lvlib\\400134"(w359) -> ()  [unwired: 1 in, 1 out]
      }
    }
    frame #6 {
      n225 = call "Imaq Dispose"("Image"=w839, "error in (no error)"=w840) -> ()  [unwired: 4 in, 1 out]
      n226 = call "Imaq Dispose"("Image"=w841, "error in (no error)"=w842) -> ()  [unwired: 4 in, 1 out]
      n227 = call <vilib>:"IMAQdx Close Camera.vi"("error in"=w843, "Session In"=w844) -> ("error out"=w838:errorcluster)  [unwired: 9 in]
      n228 = call-poly <vilib>:"Undeploy Libraries.vi"("library path"=w834) -> ("error out"=w836:errorcluster)  [unwired: 8 in]
      n229 = call <vilib>:"IMAQdx Close Camera.vi"("error in"=w838, "Session In"=w837) -> ()  [unwired: 9 in, 1 out]
      n230 = Merge Errors(w836) -> (→"Error Out":errorcluster)
    }
  }
